vi "IconModifier.vi"() -> ()   [LabVIEW 2013]
uses:
  <userlib>/_OpenG.lib/file/file.llb/File Exists - Scalar__ogtk.vi
panel:
  in  "Arguments":string[](array[string])=["--path", "<path to \"Icon Test VI\" here>", "--lines", "icon line1;icon line2;line3;line4"]
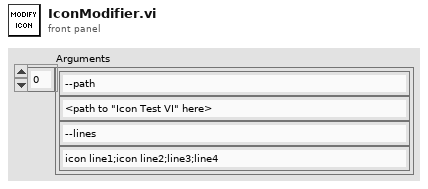
[diagram p1: front panel]
types:
  T1 = typedef "BodyText.ctl" = cluster{"Line 1 text":string, "Line 2 text":string, "Line 3 text":string, "Line 4 text":string, "Line 1 color":u32, "Line 2 color":u32, "Line 3 color":u32, "Line 4 color":u32, "Body Text Spec":cluster{"Font":T2, "Alignment":T3, "Size":u8}, "Center text vertically":bool, "Capitalize Text":bool}
  T2 = typedef "Font.ctl" = string
  T3 = typedef "Alignment.ctl" = u16
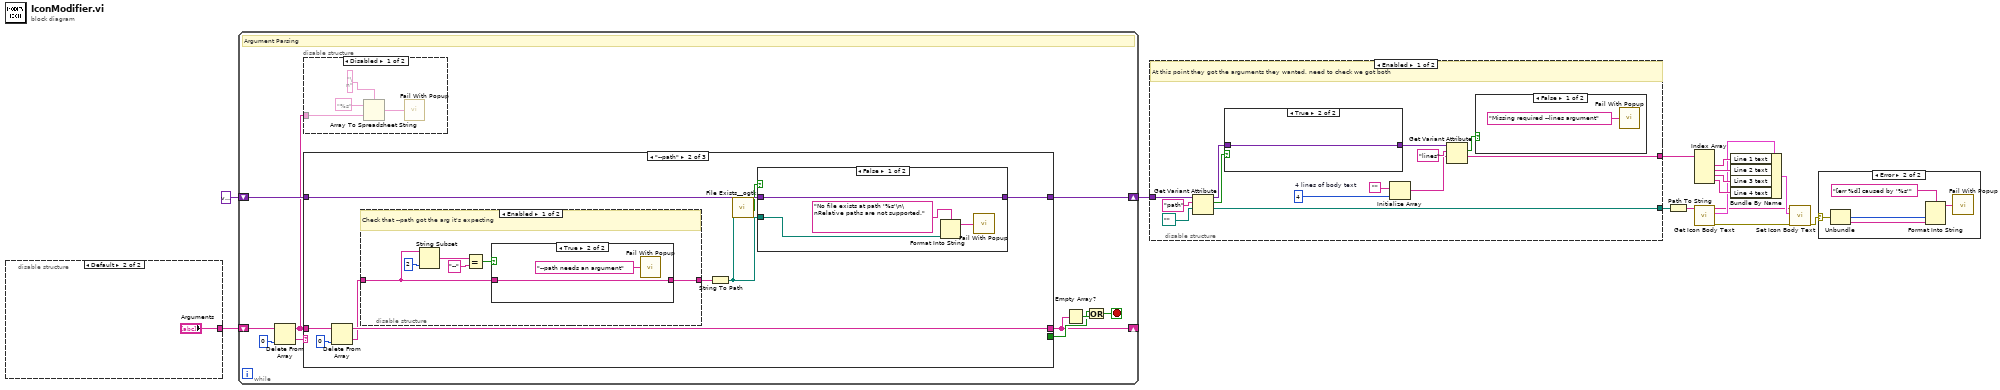
[diagram p0: block diagram]
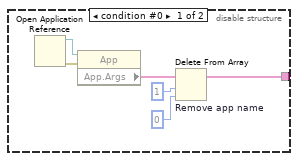
[diagram p2: hidden frame]
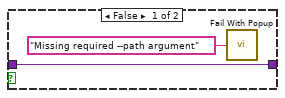
[diagram p5: hidden frame]
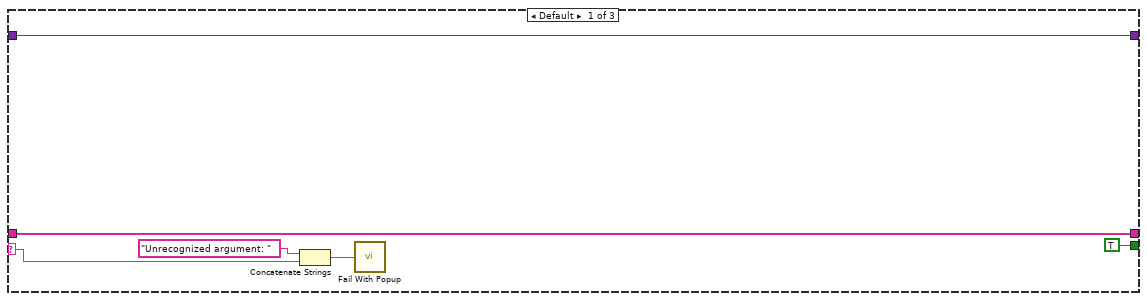
[diagram p8: hidden frame]
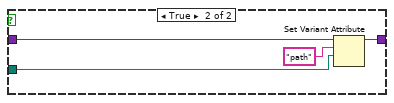
[diagram p11: hidden frame]
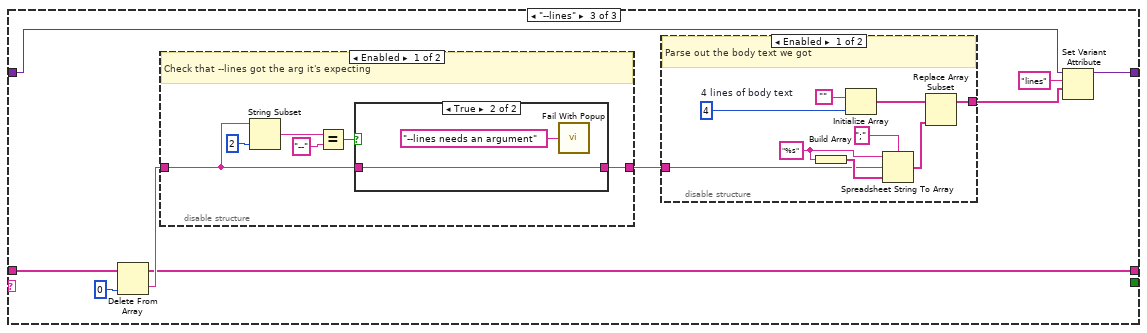
[diagram p12: hidden frame]
diagram:
  n1 = disable-structure shown="Default" {
    disable-tunnel: [w19 "Arguments"] -> w5
    frame condition #0 {
      n2 = Open Application Reference() -> (0:w20:errorcluster, 3:w21:refnum<vi>)  [unwired: 4 in]
      n3 = property class="App"(reference=w21, error in=w20) -> ("App.Args"=w16:string[])  [unwired: 2 out]
      n4 = Delete From Array "Remove app name"(array=w16, length=1, index=0) -> (array with subset deleted=w19:string[])  [unwired: 1 out]
    }
    frame condition #1 (active) {
    }
  }
  n5 = while {
    shift-right: [w26] -> _
    shift-left: w5 -> [w32]
    shift-right: [w31] -> w14
    shift-left: variant ("variant") -> [w30]
    stop <- w29 stop-if-true
    # "Argument Parsing"
    n6 = Delete From Array(array=w32, index=0) -> (deleted portion=w23:string, array with subset deleted=w25:string[])  [unwired: 1 in]
    n7 = disable-structure shown="Disabled" {
      disable-tunnel: w25 -> [w33 _]
      frame Disabled {
        n8 = Array To Spreadsheet String(delimiter (Tab)="\n", array=w33, 3:"%s" ("format string")) -> (spreadsheet string=w35:string)
        n9 = call "Fail With Popup.vi"("String"=w35) -> ()  [unwired: 1 in]
      }
      frame Enabled {
      }
    }
    n10 = case shown="\"--path\"" w23 {
      selector: w23 -> [w39 _ _]
      tunnel: [TRUE _ _] -> w27
      tunnel: [w41 w50 w70] -> w26
      tunnel: w25 -> [w41 w51 w77]
      tunnel: [w37 w48 w73] -> w31
      tunnel: w30 -> [w37 w49 w74]
      frame Default {
        n11 = Concatenate Strings("Unrecognized argument: " ("message"), w39) -> (w38:string)
        n12 = call "Fail With Popup.vi"("String"=w38) -> ()  [unwired: 1 in]
      }
      frame "--path" {
        n13 = Delete From Array(array=w51, index=0) -> (deleted portion=w45:string, array with subset deleted=w50:string[])  [unwired: 1 in]
        n14 = disable-structure shown="Enabled" {
          disable-tunnel: w45 -> [w53 _]
          disable-tunnel: [w52 _] -> w43
          frame Enabled {
            # "Check that --path got the arg it's expecting"
            n15 = String Subset(string=w53, length (rest)=2 ("length (rest)")) -> (substring=w56:string)  [unwired: 1 in]
            n16 = Equal?(x=w56, y="--") -> (x = y?=w54:bool)
            n17 = case shown="True" w54 {
              tunnel: w53 -> [w58 w59]
              tunnel: [w58 w59] -> w52
              frame False {
              }
              frame True {
                n18 = call "Fail With Popup.vi"("String"="--path needs an argument") -> ()  [unwired: 1 in]
              }
            }
          }
          frame Disabled {
          }
        }
        n19 = String To Path(string=w43) -> (path=w46:path)
        n20 = call-poly <userlib>:"File Exists__ogtk.vi"("file path"=w46) -> ("exists"=w47:bool)  [unwired: 6 in, 1 out]
        n21 = case shown="False" w47 {
          tunnel: w49 -> [w61 w68]
          tunnel: [w61 w67] -> w48
          tunnel: w46 -> [w63 w65]
          frame False {
            n22 = Format Into String(format string="No file exists at path '%s'\n\nRelative paths are not supported.", w63) -> (resulting string=w62:string)  [unwired: 2 in, 1 out]
            n23 = call "Fail With Popup.vi"("String"=w62) -> ()  [unwired: 1 in]
          }
          frame True {
            n24 = Set Variant Attribute(Variant=w68, name="path", value=w65) -> (Variant out=w67:variant)  [unwired: 1 in, 2 out]
          }
        }
      }
      frame "--lines" {
        n25 = Delete From Array(array=w77, index=0) -> (deleted portion=w76:string, array with subset deleted=w70:string[])  [unwired: 1 in]
        n26 = disable-structure shown="Enabled" {
          disable-tunnel: w76 -> [w88 _]
          disable-tunnel: [w87 _] -> w75
          frame Enabled {
            # "Check that --lines got the arg it's expecting"
            n27 = String Subset(string=w88, length (rest)=2 ("length (rest)")) -> (substring=w91:string)  [unwired: 1 in]
            n28 = Equal?(x=w91, y="--") -> (x = y?=w89:bool)
            n29 = case shown="True" w89 {
              tunnel: w88 -> [w93 w94]
              tunnel: [w93 w94] -> w87
              frame False {
              }
              frame True {
                n30 = call "Fail With Popup.vi"("String"="--lines needs an argument") -> ()  [unwired: 1 in]
              }
            }
          }
          frame Disabled {
          }
        }
        n31 = disable-structure shown="Enabled" {
          disable-tunnel: w75 -> [w79 _]
          disable-tunnel: [w78 _] -> w71
          frame Enabled {
            w82 = 4  # 4 lines of body text
            w85 = "%s" ("format string")
            # "Parse out the body text we got"
            n32 = Build Array(w85) -> (w84:string[])
            n33 = Initialize Array("", w82) -> (w81:string[])
            n34 = Spreadsheet String To Array(delimiter (Tab)=";", format string=w85, spreadsheet string=w79, array type (2D Dbl)=w84) -> (array=w80:string[])
            n35 = Replace Array Subset(array=w81, new element=w80) -> (w78:string[])  [unwired: 1 in]
          }
          frame Disabled {
          }
        }
        n36 = Set Variant Attribute(Variant=w74, name="lines", value=w71) -> (Variant out=w73:variant)  [unwired: 1 in, 2 out]
      }
    }
    n37 = Empty Array?(array=w26) -> (empty?=w28:bool)
    n38 = Or(x=w27, y=w28) -> (x .or. y?=w29:bool)
  }
  n39 = disable-structure shown="Enabled" {
    disable-tunnel: w14 -> [w108 _]
    disable-tunnel: [w97 _] -> w13
    disable-tunnel: [w96 _] -> w11
    frame Enabled {
      w103 = 4  # 4 lines of body text
      # "At this point they got the arguments they wanted, need to check we got both"
      n40 = Get Variant Attribute(Variant=w108, name="path", default value (empty Variant)=path "") -> (duplicate Variant=w99:variant, found=w105:bool, value=w97:path)  [unwired: 1 in, 1 out]
      n41 = case shown="True" w105 {
        tunnel: [w110 w112] -> w100
        tunnel: w99 -> [w110 w112]
        frame False {
          n42 = call "Fail With Popup.vi"("String"="Missing required --path argument") -> ()  [unwired: 1 in]
        }
        frame True {
        }
      }
      n43 = Initialize Array("", w103) -> (w101:string[])
      n44 = Get Variant Attribute(Variant=w100, name="lines", default value (empty Variant)=w101) -> (found=w98:bool, value=w96:string[])  [unwired: 1 in, 2 out]
      n45 = case shown="False" w98 {
        frame False {
          n46 = call "Fail With Popup.vi"("String"="Missing required --lines argument") -> ()  [unwired: 1 in]
        }
        frame True {
        }
      }
    }
    frame Disabled {
    }
  }
  n47 = Path To String(path=w13) -> (string=w2:string)
  n48 = Index Array(array=w11) -> (element #1=w10:string, element #2=w9:string, element #3=w8:string, element #4=w7:string)  [unwired: 4 in]
  n49 = call "Get Icon Body Text.vi"("VI Path"=w2) -> ("error out"=w4:errorcluster, "Body Text"=w3:T1, "VI Path (dup)"=w1:string)  [unwired: 8 in]
  n50 = Bundle By Name(cluster=w3, "Line 1 text"=w10, "Line 2 text"=w9, "Line 3 text"=w8, "Line 4 text"=w7) -> (w12:T1)
  n51 = call "Set Icon Body Text.vi"("error in (no error)"=w4, "Body Text"=w12, "VI Path"=w1) -> ("error out"=w6:errorcluster)  [unwired: 8 in]
  n52 = case shown="Error" w6 {
    selector: w6 -> [_ w117]
    frame No Error {
    }
    frame Error {
      n53 = Unbundle(w117) -> ("code"=w115:i32, "source"=w114:string)  [unwired: 1 out]
      n54 = Format Into String(format string="[err %d] caused by '%s'", w115, w114) -> (resulting string=w113:string)  [unwired: 2 in, 1 out]
      n55 = call "Fail With Popup.vi"("String"=w113) -> ()  [unwired: 1 in]
    }
  }
